vi "Calculate switch settings.vi"(0 "Plant  state":u16(ring)=1) -> (2 "Plant State out":u16(ring)=1, 3 "fractions":dbl[](array[numeric]), 4 "Control error":errorcluster[](array[cluster]))   [LabVIEW 2010]
uses:
  logic buffer cmd.ctl
  DAQ configuration/Sensor buffer command.ctl
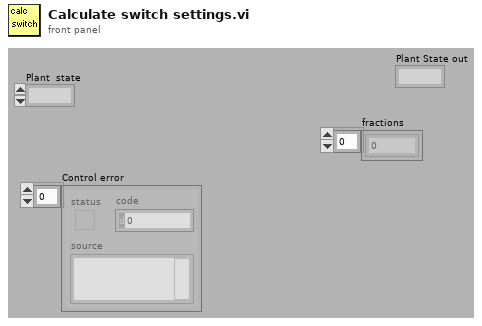
[diagram p1: front panel]
types:
  T1 = typedef "logic buffer cmd.ctl" = enum16{"read", "write ouput settings", "write rules", "write setpoints", "write output descriptions", "write all", "calculate setpoints", "save", "open", "Load all setpoint code", "Load one setpoint code"}
  T2 = typedef "variable setpoint.ctl" = cluster{"name":string, "unit":string, "value":dbl, "Type":enum16{"Constant", "Variable"}, "variable":cluster{"selected sensors":i32[], "selected set points":i32[], "VI":path, "Data average interval":T3, "code ref":T4}}
  T3 = typedef "data ave interval.ctl" = dbl
  T4 = typedef "type specifier for control code.ctl" = refnum<vi>
  T5 = typedef "Output control.ctl" = u16[][]
  T6 = typedef "Sensor buffer command.ctl" = enum16{"read average", "read recent", "read all", "write", "configure", "clear"}
  T7 = typedef "Sensor data.ctl" = cluster{" Sensor array":T8[], "Time":dbl}
  T8 = typedef "sensor cluster.ctl" = cluster{"voltage":sgl, "scaled":sgl, "units":string, "Out of Range":bool}
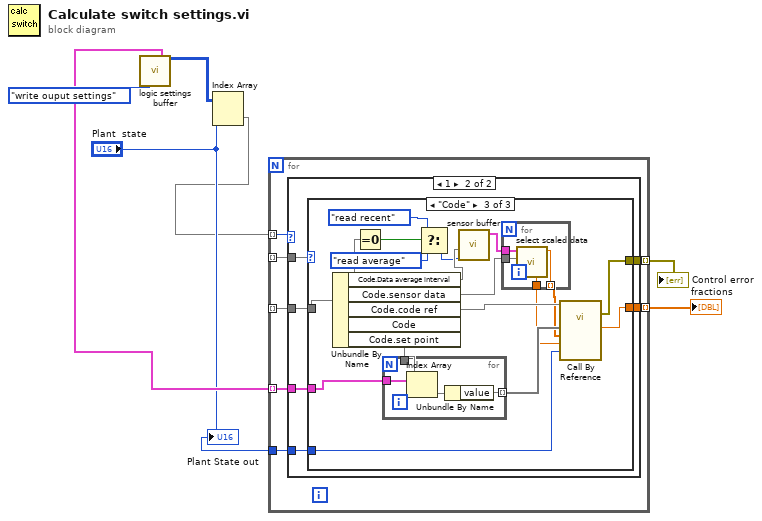
[diagram p0: block diagram]
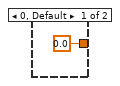
[diagram p2: hidden frame]
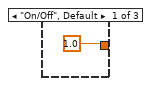
[diagram p3: hidden frame]
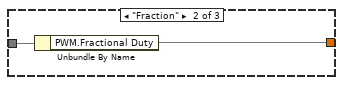
[diagram p4: hidden frame]
diagram:
  n1 = call "logic settings buffer.vi"("command"=logic_buffer_cmd."write ouput settings") -> ("Set Points out"=w5:T2[], "ouput settings out"=w2:T5)  [unwired: 10 in, 3 out]
  n2 = Index Array(array=w2, index (row)="Plant  state") -> (element=w1:u16[])  [unwired: 1 in]
  n3 = for {
    tunnel: w1 -> [w14] mode=indexing
    tunnel: _ -> [w13] mode=indexing
    tunnel: _ -> [w12] mode=indexing
    tunnel: [w11] -> w7 mode=indexing
    tunnel: w5 -> [w10] mode=indexing
    tunnel: [w9] -> w4 mode=indexing
    tunnel: "Plant  state" -> [w8]
    n4 = case shown="1" w14 {
      tunnel: w13 -> [_ w20]
      tunnel: w12 -> [_ w21]
      tunnel: [0.0 ("Fractional Duty") w19] -> w11
      tunnel: w10 -> [_ w18]
      tunnel: [_ w17] -> w9
      tunnel: w8 -> [_ w16]
      frame 0, Default {
      }
      frame 1 {
        n5 = case shown="\"Code\"" w21 {
          tunnel: w20 -> [_ w24 w41]
          tunnel: [1.0 w23 w34] -> w19
          tunnel: w18 -> [_ _ w30]
          tunnel: [_ _ w27] -> w17
          tunnel: w16 -> [_ _ w25]
          frame "On/Off", Default {
          }
          frame "Fraction" {
            n6 = Unbundle By Name(w24) -> ("PWM.Fractional Duty"=w23)
          }
          frame "Code" {
            n7 = Unbundle By Name(w41) -> ("Code.Data average interval"=w32, "Code.sensor data"=w37, "Code.code ref"=w40, "Code.set point"=w39)  [unwired: 1 out]
            n8 = Equal To 0?(x=w32) -> (x = 0?=w33:bool)
            n9 = for {
              tunnel: w39 -> [w49]
              tunnel: [w47] -> w36 mode=indexing
              tunnel: w30 -> [w46]
              n10 = Index Array(array=w46, index=w49) -> (element=w48)
              n11 = Unbundle By Name(w48) -> ("value"=w47)
            }
            n12 = Select(t=Sensor_buffer_command."read recent" ("command"), s=w33, f=Sensor_buffer_command."read average" ("command")) -> (s? t:f=w31:T6)
            n13 = call "sensor buffer.vi"("command"=w31, "smooth interval (s)"=w32) -> ("Sensor Data smoothed"=w38:T7)  [unwired: 3 in, 2 out]
            n14 = for {
              tunnel: w38 -> [w45]
              tunnel: w37 -> [w44]
              tunnel: [w43] -> w26 mode=indexing
              tunnel: [w42] -> w35
              n15 = call "select scaled data.vi"("Sensor index"=w44, "Sensor Data"=w45) -> ("scaled"=w43:sgl, "Time"=w42:dbl)  [unwired: 4 in, 4 out]
            }
            n16 = call-by-ref "?"(reference=w40, "State"=w25, "Time"=w35, "Sensor Values"=w26, "Set Points"=w36) -> (error out=w27:errorcluster, "fraction on"=w34:dbl)  [unwired: 3 in, 2 out]
          }
        }
      }
    }
  }
  "fractions" <- w7
  "Control error" <- w4
  "Plant State out" <- "Plant  state"
